vi "Template - Queue2.vi"(7 "Queue Selector":T3=enum."EnQ", 8 "error in (no error)":errorcluster, 10 "Queue Data":cluster{"Enum":T2, "Variant":variant}) -> (0 "error out":errorcluster, 2 "Queue Data (out)":cluster{"Enum":T2, "Variant":variant}, 3 "Q2 Ref":T1)   [LabVIEW 2012]
uses:
  Navistar Library/Controls/TypeDef - Queue Selector(Standard).ctl
  TypeDef - Template - Queue2 Data Enum.ctl
  TypeDef - Template - Q2 Ref.ctl
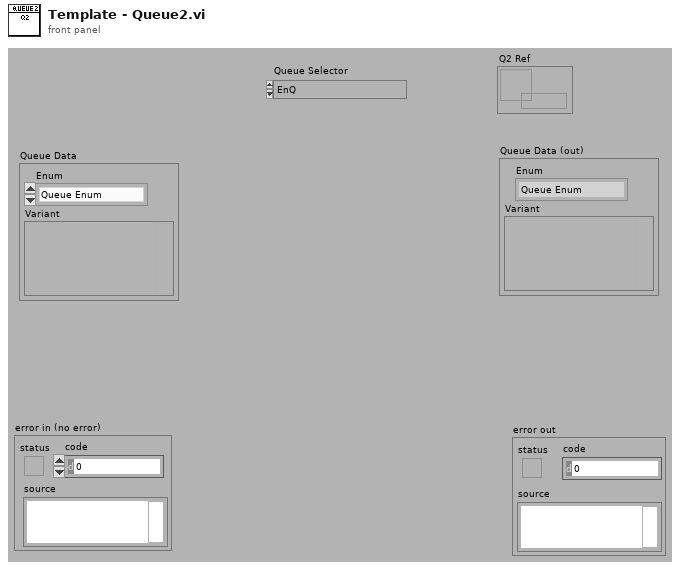
[diagram p1: front panel]
types:
  T1 = typedef "TypeDef - Template - Q2 Ref.ctl" = refnum<queue>
  T2 = typedef "TypeDef - Template - Queue2 Data Enum.ctl" = enum16{"Queue Enum", "Change RPM", "Stop"}
  T3 = typedef "TypeDef - Queue Selector(Standard).ctl" = enum16{"Create Q", "EnQ", "EnQ at the Opposite", "Flush Q", "Get Q Ref", "Clear Q", "Reset Q"}
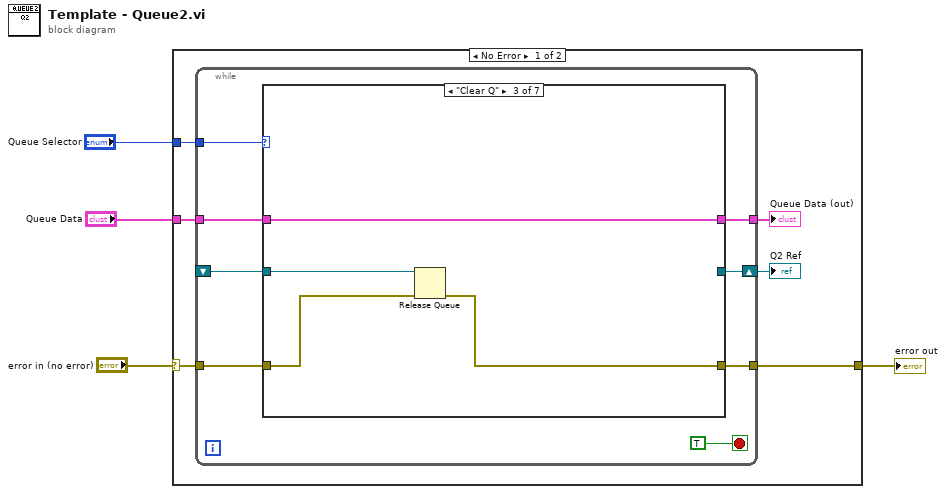
[diagram p0: block diagram]
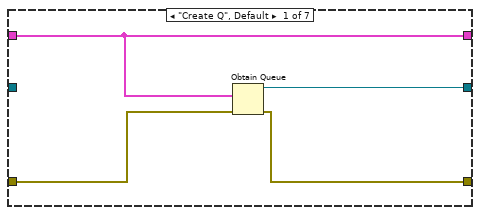
[diagram p2: hidden frame]
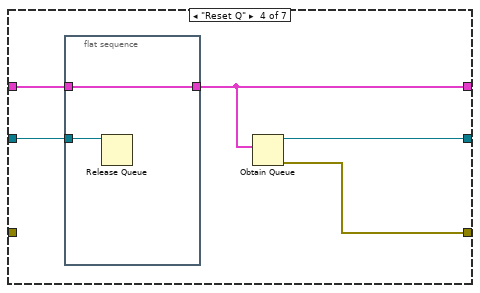
[diagram p4: hidden frame]
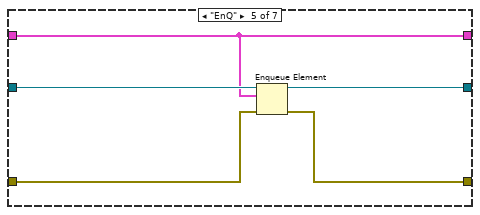
[diagram p5: hidden frame]
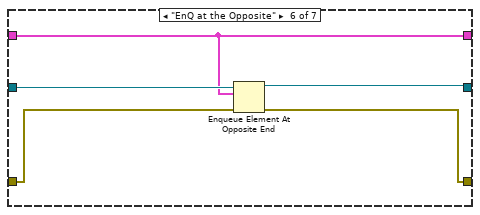
[diagram p6: hidden frame]
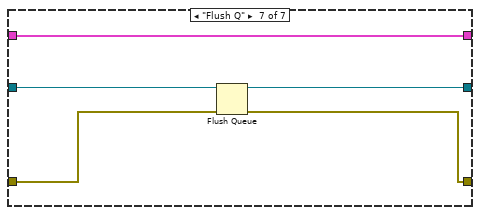
[diagram p7: hidden frame]
diagram:
  n1 = case shown="No Error" "error in (no error)" {
    selector: "error in (no error)" -> [w10 w52]
    tunnel: [w9 w52] -> w3
    tunnel: "Queue Selector" -> [w8 _]
    tunnel: "Queue Data" -> [w7 _]
    frame No Error {
      n2 = while {
        shift-right: [w18] -> w5
        shift-left: _ -> [w15]
        tunnel: w10 -> [w17]
        tunnel: [w16] -> w9
        tunnel: w7 -> [w12]
        tunnel: w8 -> [w14]
        tunnel: [w11] -> w6
        stop <- TRUE stop-if-true
        n3 = case shown="\"Clear Q\"" w14 {
          tunnel: [w21 w25 _ w32 w40 w45 w48] -> w18
          tunnel: w17 -> [w22 w24 w27 _ w39 w44 w50]
          tunnel: [w20 w24 w29 w31 w38 w43 w49] -> w16
          tunnel: w15 -> [_ w25 w28 w34 w41 w46 w51]
          tunnel: w12 -> [w19 w23 w26 w33 w37 w42 w47]
          tunnel: [w19 w23 w26 w30 w37 w42 w47] -> w11
          frame "Create Q", Default {
            n4 = Obtain Queue(element data type=w19, error in (no error)=w22) -> (queue out=w21:refnum<queue>, error out=w20:errorcluster)  [unwired: 3 in, 1 out]
          }
          frame "Get Q Ref" {
          }
          frame "Clear Q" {
            n5 = Release Queue(queue=w28, error in (no error)=w27) -> (error out=w29:errorcluster)  [unwired: 1 in, 2 out]
          }
          frame "Reset Q" {
            n6 = flat-sequence {
              tunnel: w34 -> [w36]
              tunnel: w33 -> [w35]
              tunnel: [w35] -> w30
              frame #0 {
                n7 = Release Queue(queue=w36) -> ()  [unwired: 2 in, 3 out]
              }
            }
            n8 = Obtain Queue(element data type=w30) -> (queue out=w32:refnum<queue>, error out=w31:errorcluster)  [unwired: 4 in, 1 out]
          }
          frame "EnQ" {
            n9 = Enqueue Element(queue=w41, element=w37, error in (no error)=w39) -> (queue out=w40:refnum<queue>, error out=w38:errorcluster)  [unwired: 1 in, 1 out]
          }
          frame "EnQ at the Opposite" {
            n10 = Enqueue Element At Opposite End(queue=w46, element=w42, error in (no error)=w44) -> (queue out=w45:refnum<queue>, error out=w43:errorcluster)  [unwired: 1 in, 1 out]
          }
          frame "Flush Q" {
            n11 = Flush Queue(queue=w51, error in (no error)=w50) -> (queue out=w48:refnum<queue>, error out=w49:errorcluster)  [unwired: 1 out]
          }
        }
      }
      "Queue Data (out)" <- w6
      "Q2 Ref" <- w5
    }
    frame Error {
    }
  }
  "error out" <- w3
